vi "ReportEnd1.vi"(6 "文件重命名":bool, 7 "产品型号":string, 8 "error in (no error)":errorcluster caption="错误输入（无错误）", 10 "文件名称":string, 11 "report in":refnum<class "NI_report.lvclass"> caption="报表输入") -> (0 "error out":errorcluster caption="错误输出")   [LabVIEW 2020]
uses:
  <vilib>/Utility/NIReport.llb/NI_report.lvclass
panel:
  out "添加的路径":path
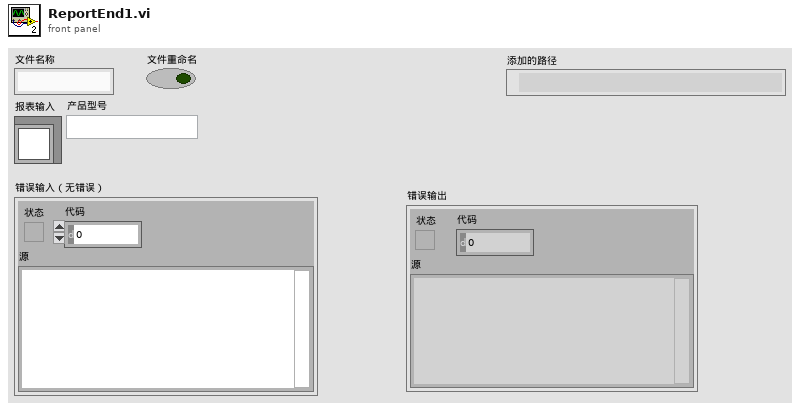
[diagram p1: front panel]
types:
  T1 = cluster{"Italic":enum16{"Italic Unchanged", "Italic On", "Italic Off"}, "Strike Through":enum16{"Strike Through Unchanged", "Strike Through On", "Strike Through Off"}, "Underline":enum16{"Underline Unchanged", "Underline On", "Underline Off"}, "Bold":enum16{"Bold Unchanged", "Bold On", "Bold Off"}}
  T2 = cluster{"Charset (-1)":i16, "Weight (-1)":i16, "Name":string, "Size":string}
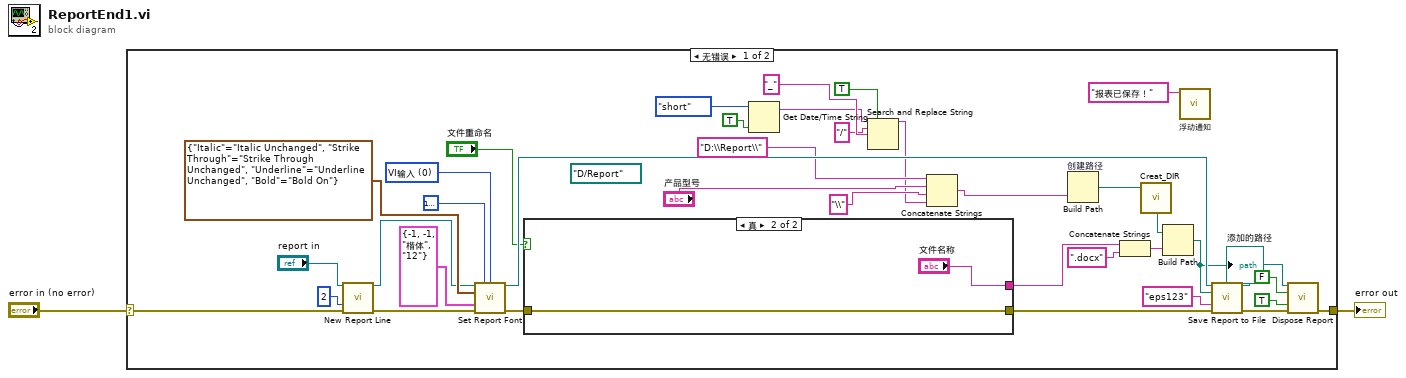
[diagram p0: block diagram]
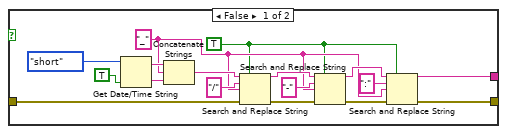
[diagram p2: hidden frame]
diagram:
  n1 = case shown="无错误" "error in (no error)" {
    selector: "error in (no error)" -> [w24 w59]
    tunnel: [w23 w59] -> w1
    frame No Error {
      w34 = u16 0 items=["VI输入", "字体对话框"] ("font settings source")
      (unwired) path "D:/Report" ("report file path")
      n2 = call-dynamic "New Report Line.vi"("report in"="report in", "number of lines (1)"=2, "error in (no error)"=w24) -> ("report out"=w31:refnum<class "NI_report.lvclass">, "error out"=w30:errorcluster)  [unwired: 11 in]
      n3 = call-dynamic "Set Report Font.vi"("report in"=w31, "text color (unchanged)"=u32 16777224, "font settings source (VI Inputs)"=w34, "text options"=T1 {"Italic"=enum."Italic Unchanged", "Strike Through"=enum."Strike Through Unchanged", "Underline"=enum."Underline Unchanged", "Bold"=enum."Bold On"}, "font settings"=T2 {"Charset (-1)"=-1, "Weight (-1)"=-1, "Name"="楷体", "Size"="12"}, "error in (no error)"=w30) -> ("report out"=w27:refnum<class "NI_report.lvclass">, "error out"=w26:errorcluster)  [unwired: 7 in, 1 out]
      n4 = case shown="真" "文件重命名" {
        tunnel: [w51 "文件名称"] -> w21
        tunnel: w26 -> [w43 w58]
        tunnel: [w40 w58] -> w25
        frame False {
          w45 = TRUE ("替换全部？(F)")
          w46 = "_" ("替换字符串(\"\")")
          n5 = Get Date/Time String(date format (0)=enum16{"short", "long", "abbreviated"}."short" ("日期格式(0)"), want seconds? (F)=TRUE ("需要秒？(F)")) -> (date string=w56:string, time string=w52:string)  [unwired: 1 in]
          n6 = Concatenate Strings(w56, w46, w52) -> (w49:string)
          n7 = Search and Replace String(replace all?=w45, input string=w49, search string="/" ("搜索字符串"), replace string=w46, error in=w43) -> (result string=w48:string, error out=w42:errorcluster)  [unwired: 3 in, 2 out]
          n8 = Search and Replace String(replace all?=w45, input string=w48, search string="-" ("搜索字符串"), replace string=w46, error in=w42) -> (result string=w54:string, error out=w41:errorcluster)  [unwired: 3 in, 2 out]
          n9 = Search and Replace String(replace all?=w45, input string=w54, search string=":" ("搜索字符串"), replace string=w46, error in=w41) -> (result string=w51:string, error out=w40:errorcluster)  [unwired: 3 in, 2 out]
        }
        frame True {
        }
      }
      n10 = Get Date/Time String(date format (0)=enum16{"short", "long", "abbreviated"}."short" ("日期格式(0)"), want seconds? (F)=TRUE ("需要秒？(F)")) -> (date string=w9:string)  [unwired: 1 in, 1 out]
      n11 = Search and Replace String(replace all?=TRUE ("替换全部？(F)"), input string=w9, search string="/" ("搜索字符串"), replace string="_" ("替换字符串(\"\")")) -> (result string=w5:string)  [unwired: 4 in, 3 out]
      n12 = Concatenate Strings("D:\\Report\\" ("字符串"), "产品型号", "\\" ("搜索字符串"), w5) -> (w4:string)
      n13 = Build Path "创建路径"(name or relative path=w4) -> (appended path=w3:path)  [unwired: 1 in]
      n14 = Concatenate Strings(w21, ".docx" ("字符串")) -> (w20:string)
      n15 = call "Creat_DIR.vi"("path"=w3) -> ("created path"=w16:path)  [unwired: 10 in]
      n16 = Build Path(base path=w16, name or relative path=w20) -> (appended path=w15:path)
      "添加的路径" <- w15
      n17 = call "浮动通知.vi"("通知内容"="报表已保存！" ("Status")) -> ()  [unwired: 11 in]
      n18 = call-dynamic "Save Report to File.vi"("report in"=w27, "report file path"=w15, "password (\"\")"="eps123" ("password (\"\")"), "error in (no error)"=w25) -> ("report out"=w39:refnum<class "NI_report.lvclass">, "error out"=w38:errorcluster)  [unwired: 10 in]
      n19 = call-dynamic "Dispose Report.vi"("report in"=w39, "wait until printing completed? (T)"=FALSE, "save changes? (F)"=TRUE, "error in (no error)"=w38) -> ("error out"=w23:errorcluster)  [unwired: 11 in]
    }
    frame Error {
    }
  }
  "error out" <- w1
